vi "Check.vi"(8 "error in (no error)":errorcluster) -> (0 "error out":errorcluster, 2 "enabled":bool)   [LabVIEW 2017, in "RTProtocol.lvlib"]
uses:
  <vilib>/addons/InsightCM/Utilities/Security/RTProtocol/RTProtocol.lvlib
  <vilib>/Utility/config.llb/Read Key (Boolean).vi
  <vilib>/Utility/config.llb/NI_LVConfig.lvlib
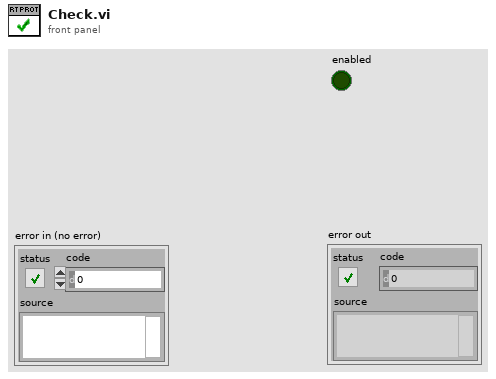
[diagram p1: front panel]
types:
  T1 = typedef "NI_LVConfig.lvlib/Config Data RefNum.ctl" = refnum<k1>
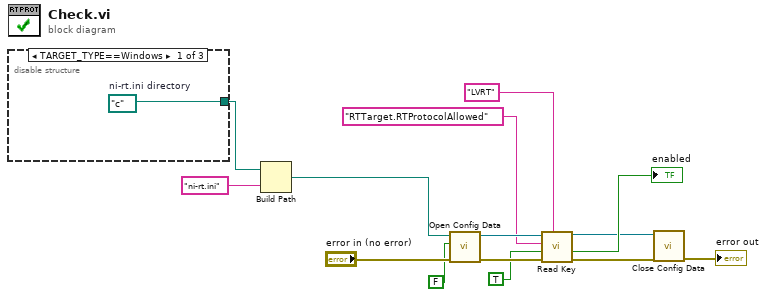
[diagram p0: block diagram]
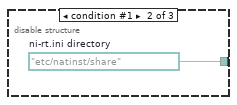
[diagram p2: hidden frame]
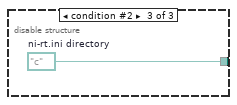
[diagram p3: hidden frame]
diagram:
  n1 = disable-structure shown="TARGET_TYPE==Windows" {
    disable-tunnel: [w15 w16 w17] -> w4
    frame condition #0 (active) {
      w15 = path "c:/"  # ni-rt.ini directory
    }
    frame condition #1 {
      w16 = path "/etc/natinst/share"  # ni-rt.ini directory
    }
    frame condition #2 {
      w17 = path "c:/"  # ni-rt.ini directory
    }
  }
  n2 = Build Path(base path=w4, name or relative path="ni-rt.ini") -> (appended path=w6:path)
  n3 = call <vilib>:"Open Config Data.vi"("error in (no error)"="error in (no error)", "create file if necessary (T)"=FALSE, "configuration file path"=w6) -> ("error out"=w13:errorcluster, "refnum"=w12:T1)  [unwired: 6 in, 1 out]
  n4 = call-poly <vilib>:"Read Key.vi"("section"="LVRT", "error in (no error)"=w13, "default value"=TRUE, "key"="RTTarget.RTProtocolAllowed", "refnum"=w12) -> ("error out"=w1:errorcluster, "value"=→"enabled":bool, "refnum out"=w3:T1)  [unwired: 3 in, 1 out]
  n5 = call <vilib>:"Close Config Data.vi"("error in (no error)"=w1, "refnum"=w3) -> ("error out"=→"error out":errorcluster)  [unwired: 8 in, 1 out]
